vi "DigitalStimulusRecord.vi"(4 "Pulse Number":i32, 6 "Pulse Interval":dbl, 7 "Channel":T2(ring), 8 "Pulse Length":dbl, 9 "Number":i32, 10 "Interval":dbl, 11 "Delay":dbl) -> (2 "digital stimulus":T1)   [LabVIEW 2015]
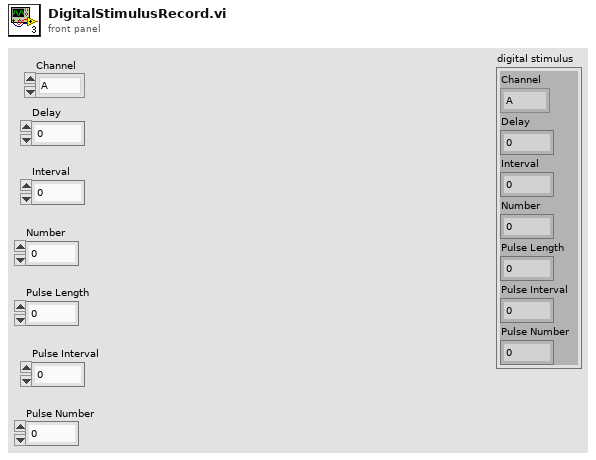
[diagram p1: front panel]
types:
  T1 = cluster{"Channel":enum16{"A", "B", "C", "D", "E", "F", "G", "H", "I", "J", "K", "L", "M", "N", "O", "P", "Q", "R", "S", "T", "U", "V", "W", "X"}, "Delay":dbl, "Interval":dbl, "Number":i32, "Pulse Length":dbl, "Pulse Interval":dbl, "Pulse Number":i32}
  T2 = enum16{"A", "B", "C", "D", "E", "F", "G", "H", "I", "J", "K", "L", "M", "N", "O", "P", "Q", "R", "S", "T", "U", "V", "W", "X"}
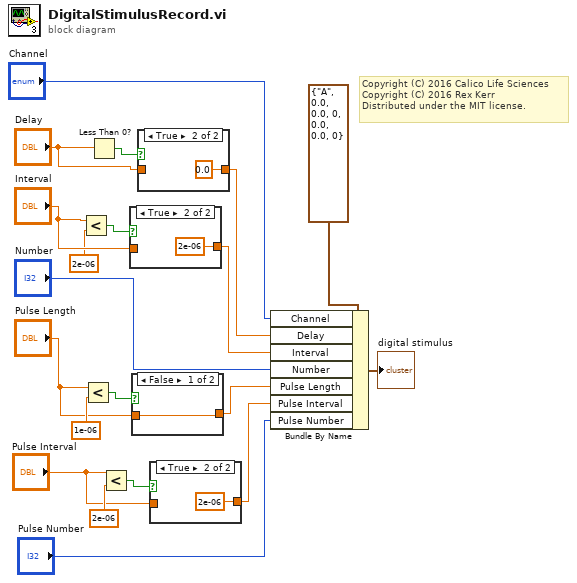
[diagram p0: block diagram]
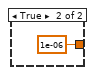
[diagram p3: hidden frame]
diagram:
  # "Copyright (C) 2016 Calico Life Sciences\nCopyright (C) 2016 Rex Kerr\nDistributed under the MIT license."
  n1 = Less?(x="Interval", y=2e-06) -> (x < y?=w12:bool)
  n2 = Less?(x="Pulse Length", y=1e-06) -> (x < y?=w8:bool)
  n3 = Less Than 0?(x="Delay") -> (x < 0?=w15:bool)
  n4 = Less?(x="Pulse Interval", y=2e-06) -> (x < y?=w4:bool)
  n5 = case shown="True" w12 {
    tunnel: [w21 2e-06 ("Delay")] -> w11
    tunnel: "Interval" -> [w21 _]
    frame False {
    }
    frame True {
    }
  }
  n6 = case shown="False" w8 {
    tunnel: [w23 1e-06 ("Delay")] -> w5
    tunnel: "Pulse Length" -> [w23 _]
    frame False {
    }
    frame True {
    }
  }
  n7 = case shown="True" w15 {
    tunnel: "Delay" -> [w25 _]
    tunnel: [w25 0.0 ("Delay")] -> w13
    frame False {
    }
    frame True {
    }
  }
  n8 = case shown="True" w4 {
    tunnel: [w27 2e-06 ("Delay")] -> w1
    tunnel: "Pulse Interval" -> [w27 _]
    frame False {
    }
    frame True {
    }
  }
  n9 = Bundle By Name(cluster=T1 {"Channel"=enum."A", "Delay"=0.0, "Interval"=0.0, "Number"=0, "Pulse Length"=0.0, "Pulse Interval"=0.0, "Pulse Number"=0}, "Channel"="Channel", "Delay"=w13, "Interval"=w11, "Number"="Number", "Pulse Length"=w5, "Pulse Interval"=w1, "Pulse Number"="Pulse Number") -> (→"digital stimulus":T1)
